vi "tEST FGV-BroadcastRegistry2.vi"() -> ()   [LabVIEW 2014]
uses:
  user.lib/_NEVSTOP/JKI State Machine ++/_Support/Typedef/_JKISM_Broadcast_ActingMsg_info.ctl
  user.lib/_NEVSTOP/JKI State Machine ++/AdvanceAPI/JKISM++ Broadcast Message Type.ctl
  user.lib/_NEVSTOP/JKI State Machine ++/_Support/FGV-BroadcastRegistry/Oper-BroadcastRegistry.ctl
  user.lib/_NEVSTOP/JKI State Machine ++/JKI-State-Machine-Plus.lvlib
panel:
  out "Cluster 10":cluster{"Registry":variant}
  out "Cluster 9":cluster{"Registry":variant}
  out "Cluster 8":cluster{"Registry":variant}
  out "ActingMsg Info":T1
  out "Cluster 7":cluster{"Registry":variant}
  out "ActingMsg Info":T1
  out "Cluster 6":cluster{"Registry":variant}
  out "Cluster 5":cluster{"Registry":variant}
  out "Cluster 4":cluster{"Registry":variant}
  out "Cluster 3":cluster{"Registry":variant}
  out "ActingMsg Info":T1
  out "Cluster 2":cluster{"Registry":variant}
  out "ActingMsg Info":T1
  out "Cluster":cluster{"Registry":variant}
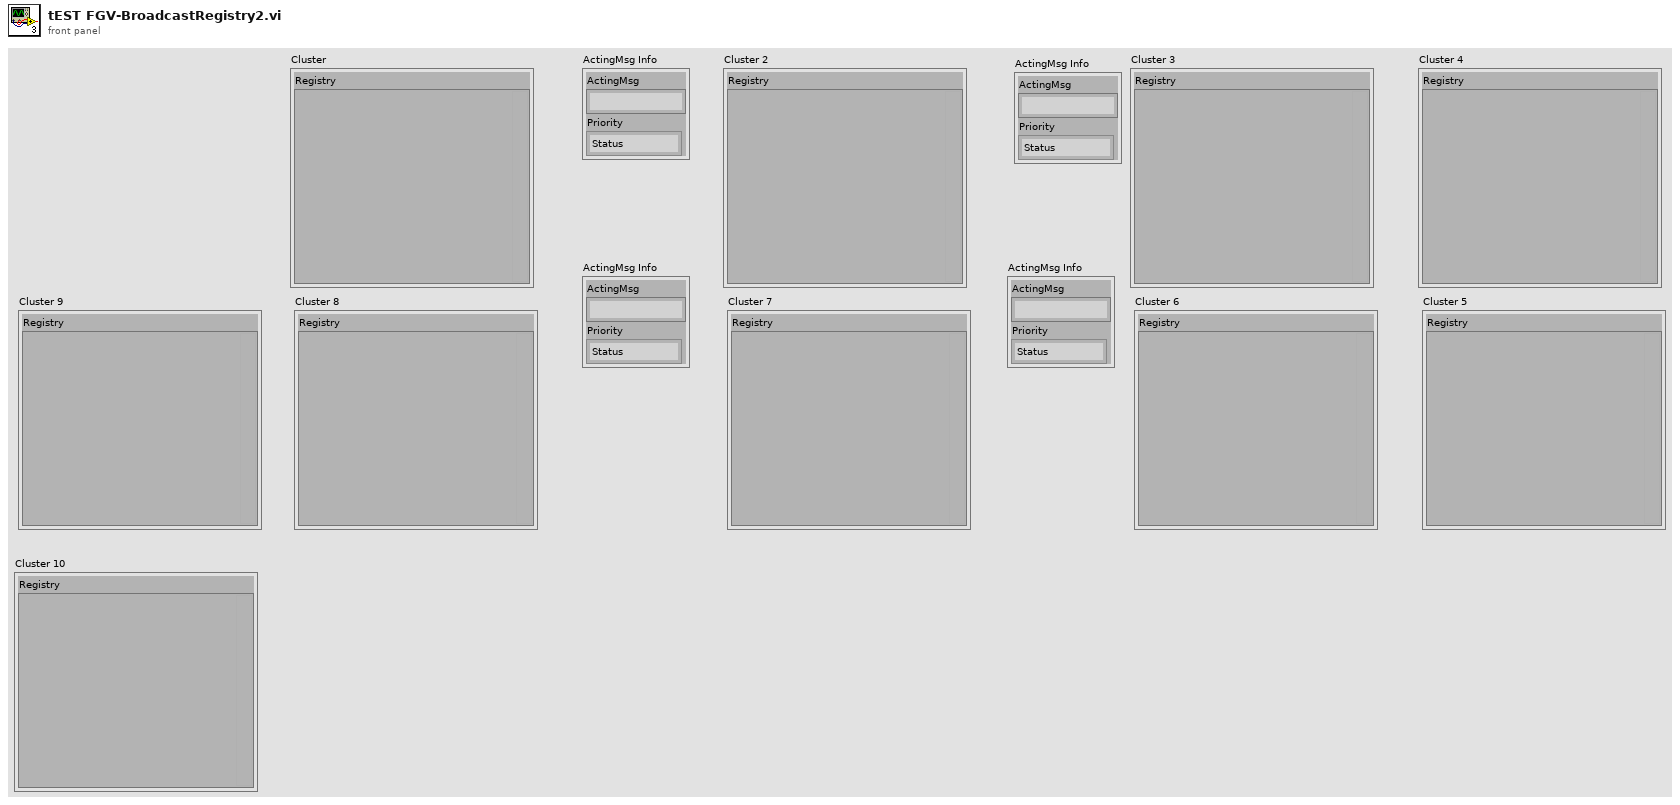
[diagram p1: front panel]
types:
  T1 = typedef "JKI-State-Machine-Plus.lvlib/_JKISM_Broadcast_ActingMsg_info.ctl" = cluster{"ActingMsg":string, "Priority":T2}
  T2 = typedef "JKI-State-Machine-Plus.lvlib/JKISM++ Broadcast Message Type.ctl" = enum16{"Status", "Interrupt(High)"}
  T3 = typedef "JKI-State-Machine-Plus.lvlib/Oper-BroadcastRegistry.ctl" = enum16{"Delete Source Module", "Delete Dest Module", "Remove Module", "Register", "Unregister", "Check"}
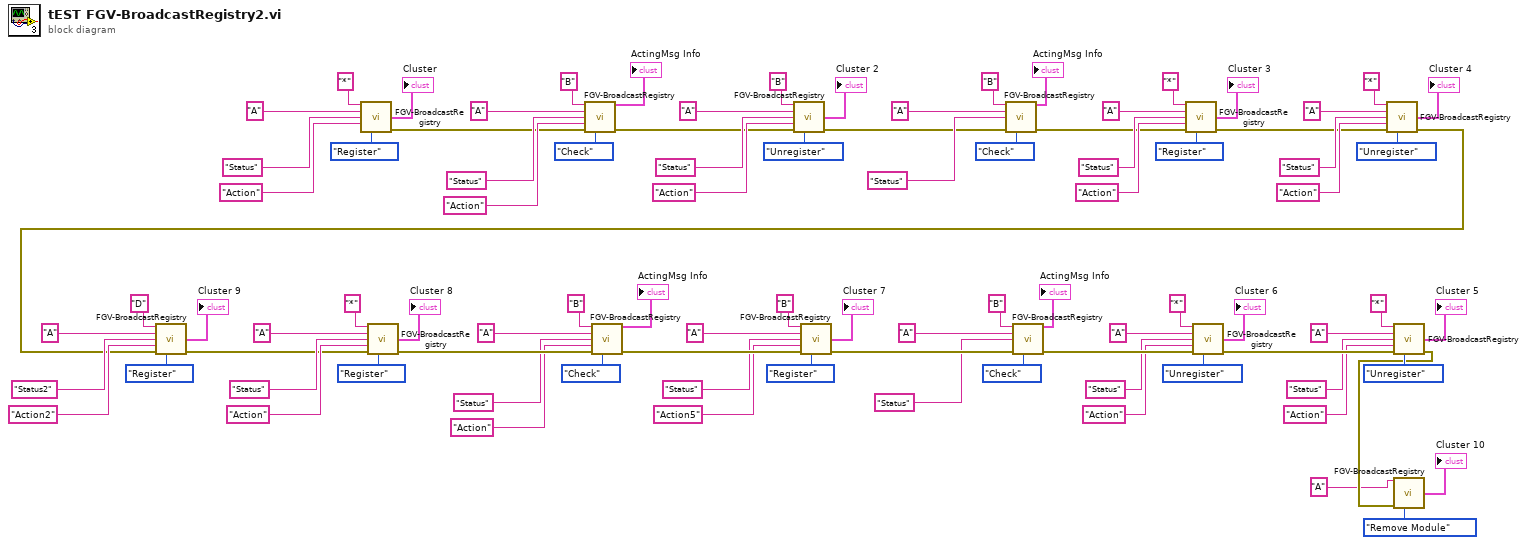
[diagram p0: block diagram]
diagram:
  n1 = call "FGV-BroadcastRegistry.vi"("Source"="*", "Dest"="A", "Message"="Status", "ActingMsg In"="Action", "Operation"=Oper-BroadcastRegistry."Register") -> ("Cluster"=→"Cluster":cluster{"Registry":variant}, "Error out"=w81:errorcluster)  [unwired: 8 in, 1 out]
  n2 = call "FGV-BroadcastRegistry.vi"("Source"="B", "Dest"="A", "Message"="Status", "ActingMsg In"="Action", "Error in"=w81, "Operation"=Oper-BroadcastRegistry."Check") -> ("ActingMsg Info"=→"ActingMsg Info":T1, "Error out"=w73:errorcluster)  [unwired: 7 in, 1 out]
  n3 = call "FGV-BroadcastRegistry.vi"("Source"="B", "Dest"="A", "Message"="Status", "ActingMsg In"="Action", "Error in"=w73, "Operation"=Oper-BroadcastRegistry."Unregister") -> ("Cluster"=→"Cluster 2":cluster{"Registry":variant}, "Error out"=w67:errorcluster)  [unwired: 7 in, 1 out]
  n4 = call "FGV-BroadcastRegistry.vi"("Source"="B", "Dest"="A", "Message"="Status", "Error in"=w67, "Operation"=Oper-BroadcastRegistry."Check") -> ("ActingMsg Info"=→"ActingMsg Info":T1, "Error out"=w60:errorcluster)  [unwired: 8 in, 1 out]
  n5 = call "FGV-BroadcastRegistry.vi"("Source"="*", "Dest"="A", "Message"="Status", "ActingMsg In"="Action", "Error in"=w60, "Operation"=Oper-BroadcastRegistry."Register") -> ("Cluster"=→"Cluster 3":cluster{"Registry":variant}, "Error out"=w53:errorcluster)  [unwired: 7 in, 1 out]
  n6 = call "FGV-BroadcastRegistry.vi"("Source"="*", "Dest"="A", "Message"="Status", "ActingMsg In"="Action", "Error in"=w53, "Operation"=Oper-BroadcastRegistry."Unregister") -> ("Cluster"=→"Cluster 4":cluster{"Registry":variant}, "Error out"=w6:errorcluster)  [unwired: 7 in, 1 out]
  n7 = call "FGV-BroadcastRegistry.vi"("Source"="D", "Dest"="A", "Message"="Status2", "ActingMsg In"="Action2", "Error in"=w6, "Operation"=Oper-BroadcastRegistry."Register") -> ("Cluster"=→"Cluster 9":cluster{"Registry":variant}, "Error out"=w5:errorcluster)  [unwired: 7 in, 1 out]
  n8 = call "FGV-BroadcastRegistry.vi"("Source"="*", "Dest"="A", "Message"="Status", "ActingMsg In"="Action", "Error in"=w5, "Operation"=Oper-BroadcastRegistry."Register") -> ("Cluster"=→"Cluster 8":cluster{"Registry":variant}, "Error out"=w24:errorcluster)  [unwired: 7 in, 1 out]
  n9 = call "FGV-BroadcastRegistry.vi"("Source"="B", "Dest"="A", "Message"="Status", "ActingMsg In"="Action", "Error in"=w24, "Operation"=Oper-BroadcastRegistry."Check") -> ("ActingMsg Info"=→"ActingMsg Info":T1, "Error out"=w32:errorcluster)  [unwired: 7 in, 1 out]
  n10 = call "FGV-BroadcastRegistry.vi"("Source"="B", "Dest"="A", "Message"="Status", "ActingMsg In"="Action5", "Error in"=w32, "Operation"=Oper-BroadcastRegistry."Register") -> ("Cluster"=→"Cluster 7":cluster{"Registry":variant}, "Error out"=w38:errorcluster)  [unwired: 7 in, 1 out]
  n11 = call "FGV-BroadcastRegistry.vi"("Source"="B", "Dest"="A", "Message"="Status", "Error in"=w38, "Operation"=Oper-BroadcastRegistry."Check") -> ("ActingMsg Info"=→"ActingMsg Info":T1, "Error out"=w45:errorcluster)  [unwired: 8 in, 1 out]
  n12 = call "FGV-BroadcastRegistry.vi"("Source"="*", "Dest"="A", "Message"="Status", "ActingMsg In"="Action", "Error in"=w45, "Operation"=Oper-BroadcastRegistry."Unregister") -> ("Cluster"=→"Cluster 6":cluster{"Registry":variant}, "Error out"=w52:errorcluster)  [unwired: 7 in, 1 out]
  n13 = call "FGV-BroadcastRegistry.vi"("Source"="*", "Dest"="A", "Message"="Status", "ActingMsg In"="Action", "Error in"=w52, "Operation"=Oper-BroadcastRegistry."Unregister") -> ("Cluster"=→"Cluster 5":cluster{"Registry":variant}, "Error out"=w2:errorcluster)  [unwired: 7 in, 1 out]
  n14 = call "FGV-BroadcastRegistry.vi"("Source"="A" ("Dest"), "Error in"=w2, "Operation"=Oper-BroadcastRegistry."Remove Module") -> ("Cluster"=→"Cluster 10":cluster{"Registry":variant})  [unwired: 10 in, 2 out]
